vi "Analogue_Input_index_array.vi"(1 "Analysis Info cluster":T1[](array[typedef]) {"Sync Delay Time (s)" format="%.4f"; "Sd Error in Variance" format="%.2f"; "Skew_u" format="%.2f"; "% u'/U" format="%.2f"; "Sd Error in Mean" format="%.2f"; "Kurt_u" format="%.2f"; "u^4" format="%.2f"; "u^3" format="%.2f"; "U" format="%.2f"; "u^2" format="%.2f"}) -> (0 "Array":i32[](array[numeric]))   [LabVIEW 2017]
uses:
  Controls/Analysis_info_cluster.ctl
  Controls/Inst_type.ctl
  Controls/Instrument_Array.ctl
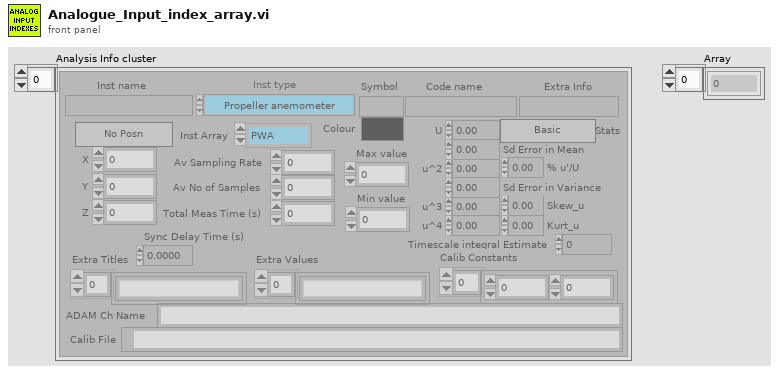
[diagram p1: front panel]
types:
  T1 = typedef "Analysis_info_cluster.ctl" = cluster{"Colour":u32, "Inst type":T2, "Inst name":string, "Symbol":string, "Code name":string, "Extra Info":string, "Inst Array":T3, "Extra Titles":string[], "Extra Values":string[], "U":dbl, "u^2":dbl, "u^3":dbl, "u^4":dbl, "Skew_u":dbl, "Kurt_u":dbl, "Sd Error in Mean":dbl, "% u'/U":dbl, "X":dbl, "Y":dbl, "Z":dbl, "Timescale integral Estimate":dbl, "Sd Error in Variance":dbl, "Calib File":path, "Calib Constants":dbl[], "Output Position":bool, "Full Stats":bool, "Av Sampling Rate":dbl, "Av No of Samples":dbl, "Total Meas Time (s)":dbl, "ADAM Ch Name":string, "Max value":dbl, "Min value":dbl, "Sync Delay Time (s)":dbl}
  T2 = typedef "Inst_type.ctl" = enum16{"Propeller anemometer", "Raw voltage", "Pressure Transducer", "Pitot-static tube", "Preston tube", "Hot wire", "Cross wire 1", "Cross wire 2", "Generic Linear", "Generic Polynomial", "Generic BackPoly", "Fast FID", "Thermocouple", "Cold wire", "Pulsed Wire", "LDA Vel", "LDA Tran time", "LDA Arr time", "Microphone"}
  T3 = typedef "Instrument_Array.ctl" = enum16{"PWA", "LDA", "Analogue"}
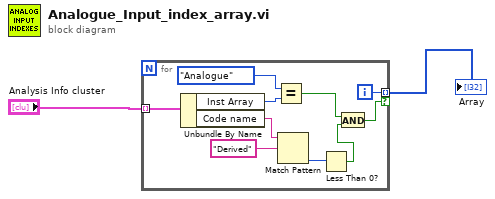
[diagram p0: block diagram]
diagram:
  n1 = for {
    tunnel: "Analysis Info cluster" -> [w5] mode=indexing
    tunnel: [w4] -> w2 mode=indexing if=w3
    i -> [w4]
    n2 = Unbundle By Name(w5) -> ("Inst Array"=w12:T3, "Code name"=w10:string)
    n3 = Equal?(x=Instrument_Array."Analogue" ("Inst Array"), y=w12) -> (x = y?=w6:bool)
    n4 = Match Pattern(string=w10, regular expression="Derived") -> (offset past match=w8:i32)  [unwired: 4 out]
    n5 = Less Than 0?(x=w8) -> (x < 0?=w7:bool)
    n6 = And(x=w6, y=w7) -> (x .and. y?=w3:bool)
  }
  "Array" <- w2
